vi "Find Direction.vi"(10 "To":T2, 11 "From":T2) -> (2 "Opposite":T1, 3 "Direction":T1, 5 "Invalid?":bool)   [LabVIEW 2020, in "Maze.lvlib" / "MazeGen.lvclass"]
uses:
  MazeGen.lvclass
  Position.ctl
  Direction.ctl
  Maze.lvlib
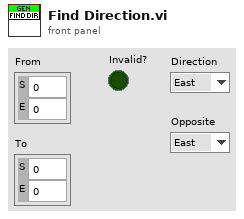
[diagram p1: front panel]
types:
  T1 = typedef "Maze.lvlib/Direction.ctl" = enum8{"East", "North", "West", "South"}
  T2 = typedef "Maze.lvlib/Position.ctl" = cluster{"S":i32, "E":i32}
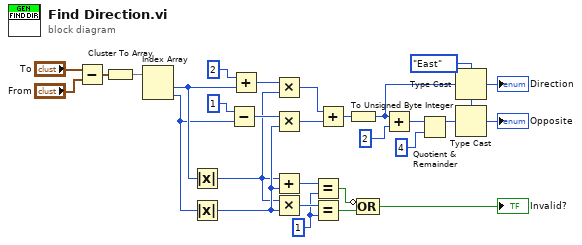
[diagram p0: block diagram]
diagram:
  w16 = 1 ("y")
  w23 = Direction."East" ("Direction")
  n1 = Subtract(x="To", y="From") -> (x-y=w20:T2)
  n2 = Cluster To Array(cluster=w20) -> (array=w19:i32[])
  n3 = Index Array(array=w19) -> (element #1=w12:i32, element #2=w8:i32)  [unwired: 2 in]
  n4 = Absolute Value(x=w12) -> (abs(x)=w2:i32)
  n5 = Absolute Value(x=w8) -> (abs(x)=w6:i32)
  n6 = Subtract(x=1, y=w8) -> (x-y=w7:i32)
  n7 = Add(x=2, y=w12) -> (x+y=w3:i32)
  n8 = Multiply(x=w3, y=w2) -> (x*y=w1:i32)
  n9 = Multiply(x=w7, y=w6) -> (x*y=w5:i32)
  n10 = Add(x=w2, y=w6) -> (x+y=w18:i32)
  n11 = Multiply(x=w2, y=w6) -> (x*y=w17:i32)
  n12 = Equal?(x=w18, y=w16) -> (x = y?=w15:bool)
  n13 = Equal?(x=w17, y=w16) -> (x = y?=w14:bool)
  n14 = Add(x=w1, y=w5) -> (x+y=w4:i32)
  n15 = To Unsigned Byte Integer(number=w4) -> (unsigned 8bit integer=w10:u8)
  n16 = Compound Arithmetic op=OR(invert w15, w14) -> (→"Invalid?":bool)
  n17 = Add(x=w10, y=u8 2) -> (x+y=w29:u8)
  n18 = Quotient & Remainder(x=w29, y=u8 4) -> (x-y*floor(x/y)=w27:u8)  [unwired: 1 out]
  n19 = Type Cast(type=w23, x=w10) -> (*(type *) &x=→"Direction":T1)
  n20 = Type Cast(type=w23, x=w27) -> (*(type *) &x=→"Opposite":T1)
